vi "Server Generate Answer Event.vi"(8 "error in":errorcluster, 10 "event data":string, 11 "server event ref":refnum<vi>) -> (0 "error out":errorcluster)   [LabVIEW 2018]
doc: "Sends answer event to server."
uses:
  <vilib>/event_ctls.llb/usereventprio.ctl
  Server Event Answer Ref.ctl
  Server Session.ctl
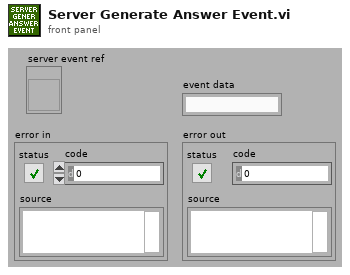
[diagram p1: front panel]
types:
  T1 = typedef "Server Session.ctl" = cluster{"cmd event":variant, "answer event":variant}
  T2 = typedef "Server Event Answer Ref.ctl" = refnum<user-event>
  T3 = typedef "usereventprio.ctl" = enum32{"high priority", "normal priority"}
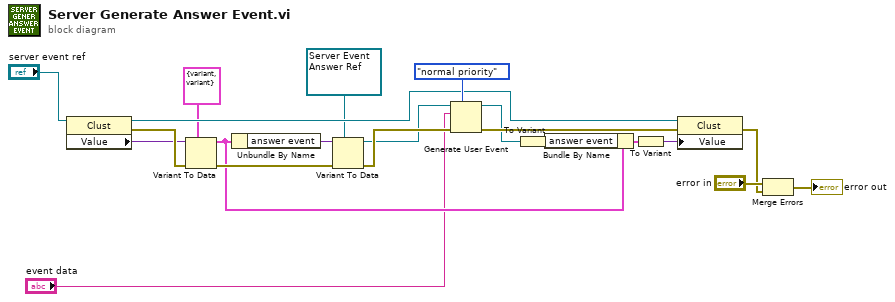
[diagram p0: block diagram]
diagram:
  n1 = property class="Clust"(reference="server event ref") -> (reference out=w19:refnum<vi>, error out=w13:errorcluster, "Value"=w12:variant)  [unwired: 1 in]
  n2 = Variant To Data(error in=w13, type=T1 {"cmd event"=variant(refnum<user-event> refnum), "answer event"=variant(refnum<user-event> refnum)} ("server"), Variant=w12) -> (data=w7:T1, error out=w11:errorcluster)
  n3 = Unbundle By Name(w7) -> ("answer event"=w9:variant)
  n4 = Variant To Data(error in=w11, type=T2 refnum ("user event out"), Variant=w9) -> (data=w16:T2, error out=w17:errorcluster)
  n5 = Generate User Event(priority (normal)=usereventprio."normal priority", user event=w16, event data cluster="event data", error in=w17) -> (user event out=w18:T2, error out=w20:errorcluster)
  n6 = To Variant(anything=w18) -> (Variant=w6:variant)
  n7 = Bundle By Name(cluster=w7, "answer event"=w6) -> (w8:T1)
  n8 = To Variant(anything=w8) -> (Variant=w5:variant)
  n9 = property class="Clust"(reference=w19, error in=w20, "Value"=w5) -> (error out=w2:errorcluster)  [unwired: 1 out]
  n10 = Merge Errors("error in", w2) -> (→"error out":errorcluster)
